vi "SerialMonitor.vi"() -> ()   [LabVIEW 2010]
panel:
  out "Response":string
  in  "Command":string
  in  "Send":bool
  # "Command:"
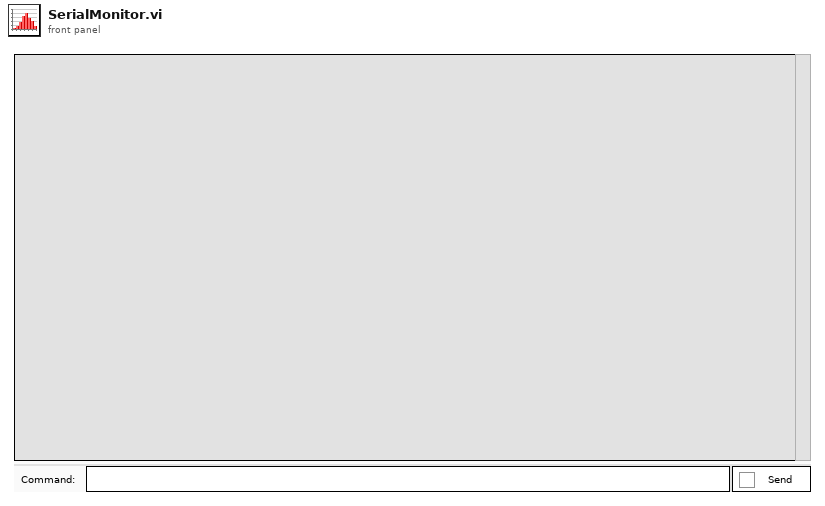
[diagram p1: front panel]
types:
  T1 = cluster{"Error":errorcluster, "GUIQueue":refnum<queue>, "TlmType":string, "NextState":string, "TextPosition":i32}
  T2 = typedef "eventvkey.ctl" = enum16{"ASCII", "Enter", "Return", "Shift", "Ctrl", "Alt", "Cmd", "Opt", "Caps", "NumLock", "Clear", "Break", "Up", "Down", "Left", "Right", "Insert", "Delete", "Home", "End", "PageUp", "PageDown", "Escape", "Help", "Pause", "ScrollLock", "F1", "F2", "F3", "F4", "F5", "F6", "F7", "F8", "F9", "F10", "F11", "F12", "F13", "F14", "F15", "F16", "F17", "F18", "F19", "F20", "F21", "F22", "F23", "F24", "Play", "VolumeUp", "VolumeDown", "Mute", "Two Byte Char"}
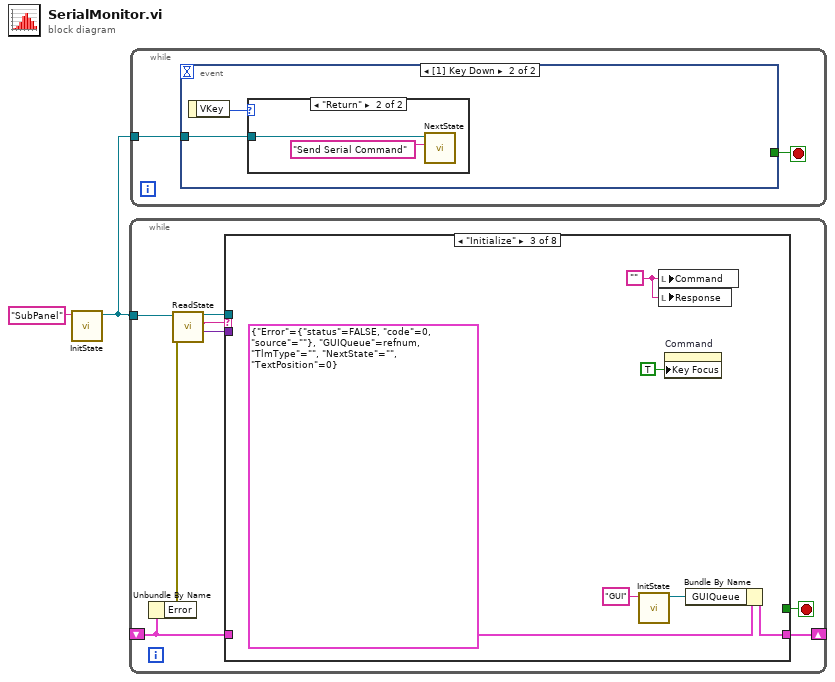
[diagram p0: block diagram]
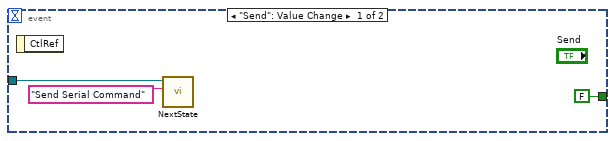
[diagram p2: hidden frame]
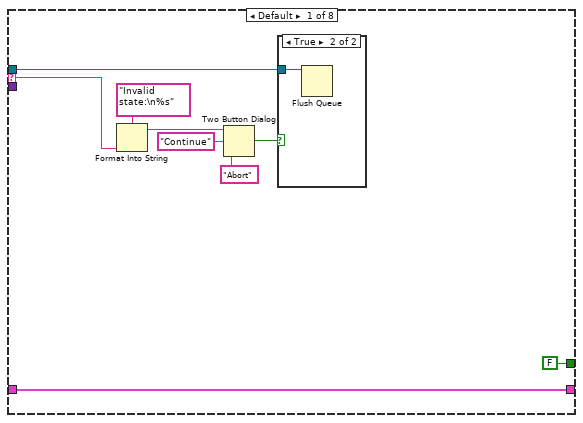
[diagram p4: hidden frame]
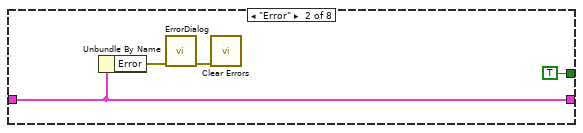
[diagram p6: hidden frame]
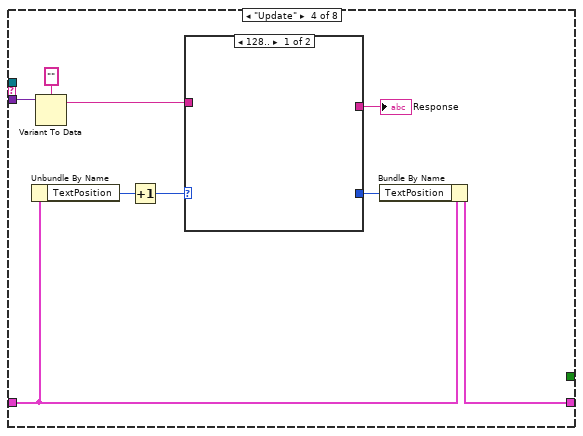
[diagram p7: hidden frame]
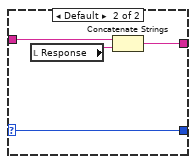
[diagram p8: hidden frame]
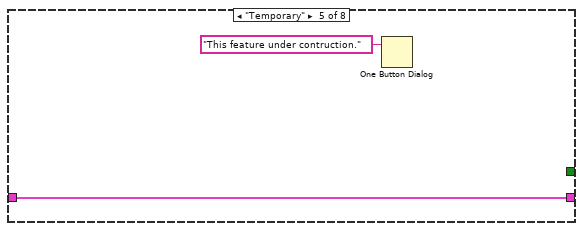
[diagram p9: hidden frame]
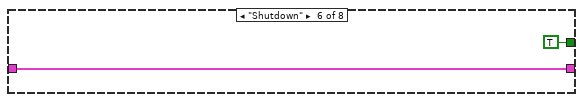
[diagram p10: hidden frame]
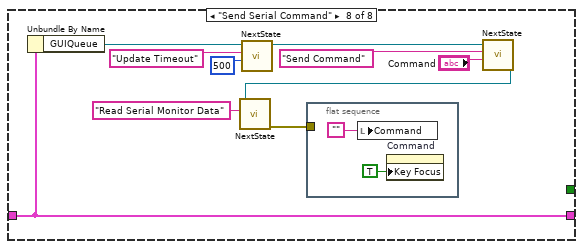
[diagram p12: hidden frame]
diagram:
  n1 = call "InitState.vi"("Name"="SubPanel" ("name (unnamed)")) -> ("Queue Out"=w1:refnum<queue>)  [unwired: 8 in, 1 out]
  n2 = while {
    tunnel: w1 -> [w7]
    shift-right: [w10] -> _
    shift-left: _ -> [w9]
    stop <- w8 stop-if-true
    n3 = Unbundle By Name(w9) -> ("Error"=w6:errorcluster)
    n4 = call "ReadState.vi"("Error In"=w6, "Queue In"=w7) -> ("Data"=w5:variant, "State"=w4:string, "Queue Out"=w3:refnum<queue>)  [unwired: 6 in, 1 out]
    n5 = case shown="\"Initialize\"" w4 {
      tunnel: w3 -> [w11 _ _ _ _ _ _ _]
      selector: w4 -> [w17 _ _ _ _ _ _ _]
      tunnel: w5 -> [_ _ _ w38 _ _ _ _]
      tunnel: [w16 w23 w29 w36 w45 w47 w48 w58] -> w10
      tunnel: w9 -> [w16 w23 _ w37 w45 w47 w48 w58]
      tunnel: [FALSE TRUE _ _ _ TRUE _ _] -> w8
      frame Default {
        n6 = Format Into String(format string="Invalid state:\n%s", w17) -> (resulting string=w18:string)  [unwired: 2 in, 1 out]
        n7 = Two Button Dialog(message=w18, 1:"Abort" ("F button name (\"Cancel\")"), 2:"Continue" ("T button name (\"OK\")")) -> (T button?=w12:bool)
        n8 = case shown="True" w12 {
          tunnel: w11 -> [_ w20]
          frame False {
          }
          frame True {
            n9 = Flush Queue(queue=w20) -> ()  [unwired: 1 in, 3 out]
          }
        }
      }
      frame "Error" {
        n10 = Unbundle By Name(w23) -> ("Error"=w22:errorcluster)
        n11 = call "ErrorDialog.vi"("error in"=w22) -> ("error out"=w21:errorcluster)  [unwired: 10 in]
        n12 = call <vilib>:"Clear Errors.vi"("error in (no error)"=w21) -> ()  [unwired: 6 in, 1 out]
      }
      frame "Initialize" {
        w26 = ""
        n13 = call "InitState.vi"("Name"="GUI") -> ("Queue Out"=w27:refnum<queue>)  [unwired: 8 in, 1 out]
        n14 = local write "Command"(w26) -> ()
        n15 = local write "Response"(w26) -> ()
        n16 = property on="Command" class="Str"("Key Focus"=TRUE) -> ()  [unwired: 2 in, 2 out]
        n17 = Bundle By Name(cluster=T1 {"Error"={"status"=FALSE, "code"=0, "source"=""}, "GUIQueue"=refnum, "TlmType"="", "NextState"="", "TextPosition"=0}, "GUIQueue"=w27) -> (w29:T1)
      }
      frame "Update" {
        n18 = Unbundle By Name(w37) -> ("TextPosition"=w33:i32)
        n19 = Variant To Data(Variant=w38, type="" ("Instruction")) -> (data=w35:string)  [unwired: 1 in, 1 out]
        n20 = Increment(x=w33) -> (x+1=w32:i32)
        n21 = case shown="128.." w32 {
          selector: w32 -> [_ w42]
          tunnel: w35 -> [_ w41]
          tunnel: [_ w43] -> w34
          tunnel: [_ w42] -> w31
          frame 128.. {
          }
          frame Default {
            n22 = local read "Response"() -> (w40:string)
            n23 = Concatenate Strings(w41, w40) -> (w43:string)
          }
        }
        "Response" <- w34
        n24 = Bundle By Name(cluster=w37, "TextPosition"=w31) -> (w36:T1)
      }
      frame "Temporary" {
        n25 = One Button Dialog(message="This feature under contruction.") -> ()  [unwired: 1 in, 1 out]
      }
      frame "Shutdown" {
      }
      frame "----------" {
      }
      frame "Send Serial Command" {
        n26 = Unbundle By Name(w58) -> ("GUIQueue"=w54:refnum<queue>)
        n27 = call "NextState.vi"("Data"=u32 500 ("General Settings:Timeout Value"), "State"="Update Timeout", "Queue In"=w54) -> ("Queue Out"=w55:refnum<queue>)  [unwired: 7 in, 1 out]
        n28 = flat-sequence {
          tunnel: w49 -> [_]
          frame #0 {
            n29 = local write "Command"("") -> ()
            n30 = property on="Command" class="Str"("Key Focus"=TRUE) -> ()  [unwired: 2 in, 2 out]
          }
        }
        n31 = call "NextState.vi"("Data"="Command", "State"="Send Command", "Queue In"=w55) -> ("Queue Out"=w51:refnum<queue>)  [unwired: 7 in, 1 out]
        n32 = call "NextState.vi"("State"="Read Serial Monitor Data", "Queue In"=w51) -> ("Error Out"=w49:errorcluster)  [unwired: 8 in, 1 out]
      }
    }
  }
  n33 = while {
    tunnel: w1 -> [w62]
    stop <- w61 stop-if-true
    n34 = event shown="[1] Key Down" {
      selector: _ -> [_ _]
      dyn-events: _ -> [_ _]
      timeout: _ -> [_ _]
      tunnel: w62 -> [w64 w66]
      tunnel: [FALSE _] -> w61
      event "Send": Value Change {
        n35 = event-data() -> ()  [unwired: 1 in, 1 out]
        n36 = call "NextState.vi"("State"="Send Serial Command", "Queue In"=w64) -> ()  [unwired: 8 in, 2 out]
      }
      event Key Down {
        n37 = event-data() -> ("VKey"=w67:T2)  [unwired: 1 in]
        n38 = case shown="\"Return\"" w67 {
          tunnel: w66 -> [_ w69]
          frame Default {
          }
          frame "Return" {
            n39 = call "NextState.vi"("State"="Send Serial Command", "Queue In"=w69) -> ()  [unwired: 8 in, 2 out]
          }
        }
      }
    }
  }
